vi "Update Previous Step Status.vi"(8 "error in (no error)":errorcluster, 10 "PreviousStep":refnum<k7>, 11 "SequenceViewPanel in":refnum<class "SequenceViewPanel.lvclass">) -> (0 "error out":errorcluster, 3 "SequenceViewPanel out":refnum<class "SequenceViewPanel.lvclass">)   [LabVIEW 2020, in "TSnax UI.lvlib" / "SequenceViewPanel.lvclass"]
uses:
  SequenceViewPanel.lvclass
  SequenceViewPanel.lvclass/SequenceViewPanel.ctl
  Step Result Request.ctl
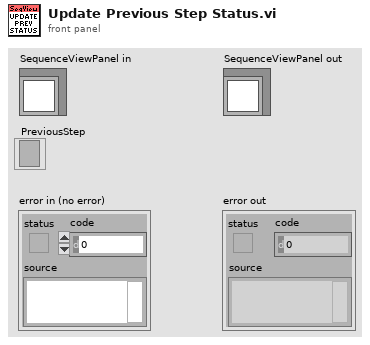
[diagram p1: front panel]
types:
  T1 = typedef "TSnax UI.lvlib/SequenceViewPanel.lvclass/Step Result Request.ctl" = cluster{"ID":string, "Result":string}
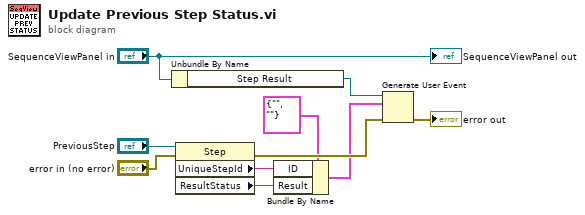
[diagram p0: block diagram]
diagram:
  n1 = Unbundle By Name("SequenceViewPanel in") -> ("Step Result"=w6:refnum<user-event>)
  n2 = property class="Step"(reference="PreviousStep", error in="error in (no error)") -> (error out=w10:errorcluster, "UniqueStepId"=w3:string, "ResultStatus"=w2:string)  [unwired: 1 out]
  n3 = Bundle By Name(cluster=T1 {"ID"="", "Result"=""} ("event data"), "ID"=w3, "Result"=w2) -> (w4:T1)
  n4 = Generate User Event(user event=w6, event data cluster=w4, error in=w10) -> (error out=→"error out":errorcluster)  [unwired: 1 in, 1 out]
  "SequenceViewPanel out" <- "SequenceViewPanel in"
